vi "Get Favorite Color.vi"(8 "error in":errorcluster, 11 "JViquez in":refnum<class "jviquez.lvclass">) -> (0 "error out":errorcluster, 2 "Favorite Color":u32(colorbox)=16777224, 3 "JViquez out":refnum<class "jviquez.lvclass">)   [LabVIEW 2023, in "JViquez.lvclass"]
uses:
  jviquez.lvclass
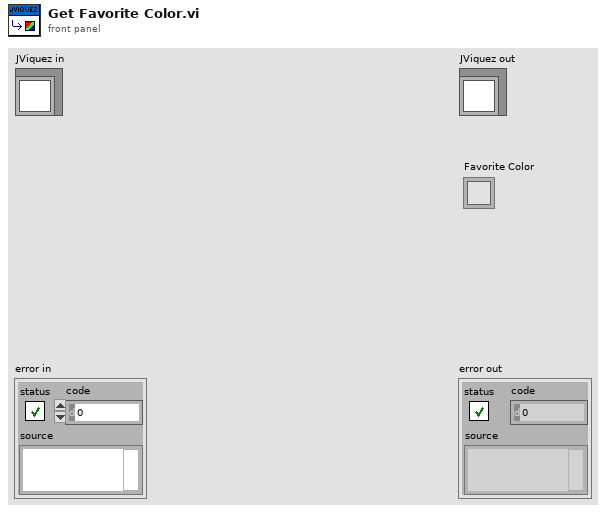
[diagram p1: front panel]
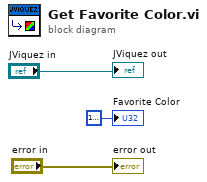
[diagram p0: block diagram]
diagram:
  "error out" <- "error in"
  "JViquez out" <- "JViquez in"
  "Favorite Color" <- u32 16777224 ("Favorite Color")
